vi "Add.vi"(8 "error in (no error)":errorcluster, 9 "parent tag":string, 10 "Destinations in":refnum<class "IB_Destination.lvclass">[](array[class]), 11 "absFolder in":refnum<class "absFolder.lvclass">) -> (0 "error out":errorcluster, 1 "duplicate?":bool, 2 "Destinations out":refnum<class "IB_Destination.lvclass">[](array[class]), 3 "absFolder out":refnum<class "absFolder.lvclass">)   [LabVIEW 2020, in "absFolder.lvclass"]
uses:
  <vilib>/AppBuilder/IB_Classes/Destination/absFolder/absFolder.lvclass
  <vilib>/AppBuilder/IB_Classes/Destination/absFolder/absFolder.lvclass/absFolder.ctl
  <vilib>/AppBuilder/IB_Classes/Destination/IB_Destination.lvclass
  e:/builds/penguin/labview/branches/2020/dev/dist/vi.lib/AppBuilder/IB_Classes/Destination/IB_Destination.lvclass
  e:/builds/penguin/labview/branches/2020/dev/dist/vi.lib/AppBuilder/IB_Classes/Destination/absFolder/absFolder.lvclass
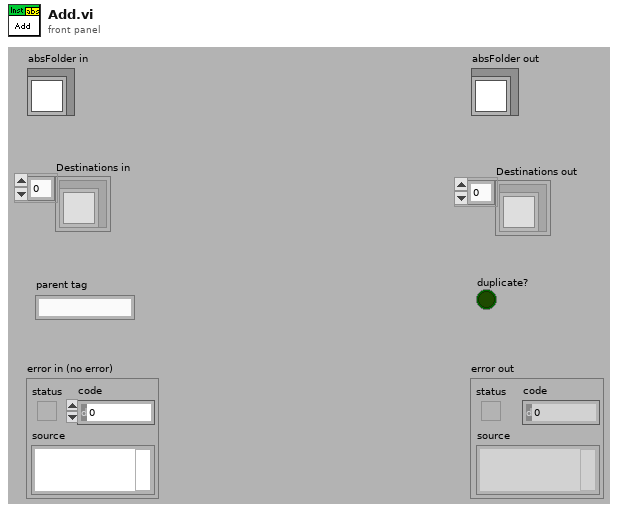
[diagram p1: front panel]
types:
  T1 = typedef "IB_Destination.ctl" = cluster{"name":string, "unlock":bool, "parentTag":string, "destTag":string, "eng_installPath":string}
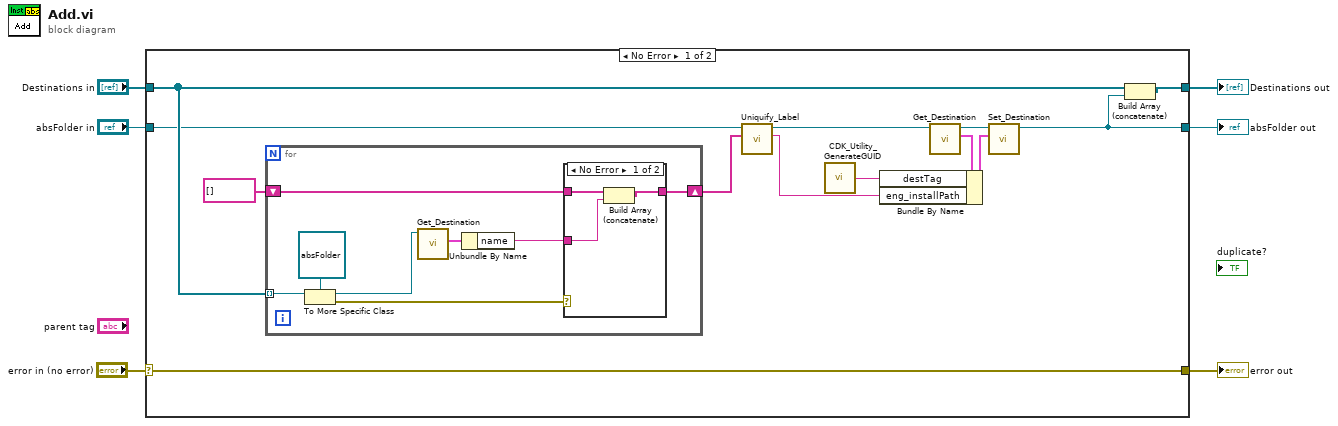
[diagram p0: block diagram]
diagram:
  n1 = case shown="No Error" "error in (no error)" {
    selector: "error in (no error)" -> [w19 w34]
    tunnel: [w19 w34] -> w5
    tunnel: "Destinations in" -> [w16 w32]
    tunnel: [w18 w32] -> w3
    tunnel: "absFolder in" -> [w15 w33]
    tunnel: [w8 w33] -> w1
    frame No Error {
      n2 = for {
        tunnel: w16 -> [w25] mode=indexing
        shift-right: [w26] -> w14
        shift-left: string[] [] -> [w27]
        n3 = To More Specific Class(target class=refnum<class "absFolder.lvclass"> refnum ("absFolder in"), reference=w25) -> (specific class reference=w22:refnum<class "absFolder.lvclass">, error out=w23:errorcluster)  [unwired: 1 in]
        n4 = call <vilib>:"Get_Destination.vi"("IB_Destination in"=w22) -> ("data"=w21:T1)  [unwired: 1 in, 9 out]
        n5 = Unbundle By Name(w21) -> ("name"=w20:string)
        n6 = case shown="No Error" w23 {
          tunnel: w27 -> [w30 w31]
          tunnel: [w29 w31] -> w26
          tunnel: w20 -> [w28 _]
          frame No Error {
            n7 = Build Array (concatenate)(w30, w28) -> (w29:string[])
          }
          frame Error {
          }
        }
      }
      n8 = call-dynamic "Uniquify_Label.vi"("names"=w14, "absFolder in"=w15) -> ("names"=w7:string, "absFolder out"=w9:refnum<class "absFolder.lvclass">)  [unwired: 1 in, 7 out]
      n9 = call <resource>:"CDK_Utility_GenerateGUID.vi"() -> ("GUID"=w13:string)  [unwired: 9 out]
      n10 = call <vilib>:"Get_Destination.vi"("IB_Destination in"=w9) -> ("data"=w11:T1, "IB_Destination out"=w12:refnum<class "absFolder.lvclass">)  [unwired: 1 in, 8 out]
      n11 = Bundle By Name(cluster=w11, "destTag"=w13, "eng_installPath"=w7) -> (w10:T1)
      n12 = call <vilib>:"Set_Destination.vi"("data"=w10, "IB_Destination in"=w12) -> ("IB_Destination out"=w8:refnum<class "absFolder.lvclass">)  [unwired: 1 in, 8 out]
      n13 = Build Array (concatenate)(w16, w8) -> (w18:refnum<class "IB_Destination.lvclass">[])
    }
    frame Error {
    }
  }
  "error out" <- w5
  "absFolder out" <- w1
  "Destinations out" <- w3
